vi "SubVI_Overlay Spot #.vi"(7 "Setup":T4={"Show Search Area"=FALSE, "Show Center"=FALSE, "Show Bounding Box"=TRUE}, 8 "Error in":errorcluster, 9 "Objects":T1(array[cluster]) {"Area" format="%.2f"; "Object Center"."Y" format="%.2f"; "Object Center"."X" format="%.2f"}, 10 "ROI":T3 {"Contours"."Type" items=["No Selection", "Point", "Line", "Rectangle", "Oval", "Polygon", "Free", "Annulus", "Unused2", "Unused3", "Broken Line", "Free Hand Line", "Rotated Rectangle"]}, 11 "Image In":T2) -> (0 "Error out":errorcluster, 3 "Image Out":T2)   [LabVIEW 2013]
uses:
  <vilib>/vision/Image Controls.llb/IMAQ Image.ctl
panel:
  in  "Center Color":u32(colorbox)=16711680
  in  "Search Area Color":u32(colorbox)=65280
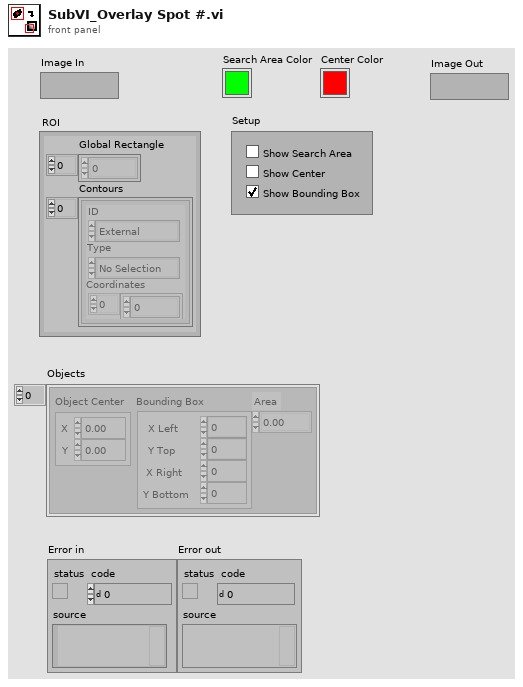
[diagram p1: front panel]
types:
  T1 = cluster{"Object Center":cluster{"X":dbl, "Y":dbl}, "Bounding Box":cluster{"X Left":dbl, "Y Top":dbl, "X Right":dbl, "Y Bottom":dbl}, "Area":dbl}[]
  T2 = typedef "IMAQ Image.ctl" = refnum<image>
  T3 = cluster{"Global Rectangle":i32[], "Contours":cluster{"ID":enum32{"External", "Internal"}, "Type":u32, "Coordinates":i32[]}[]}
  T4 = cluster{"Show Search Area":bool, "Show Center":bool, "Show Bounding Box":bool}
  T5 = cluster{"[0]":sgl, "[1]":sgl, "[2]":sgl, "[3]":sgl}
  T6 = cluster{"[0]":i32, "[1]":i32, "[2]":i32, "[3]":i32}
  T7 = cluster{"X Left":dbl, "Y Top":dbl, "X Right":dbl, "Y Bottom":dbl}
  T8 = cluster{"X Left":i32, "Y Top":i32, "X Right":i32, "Y Bottom":i32}
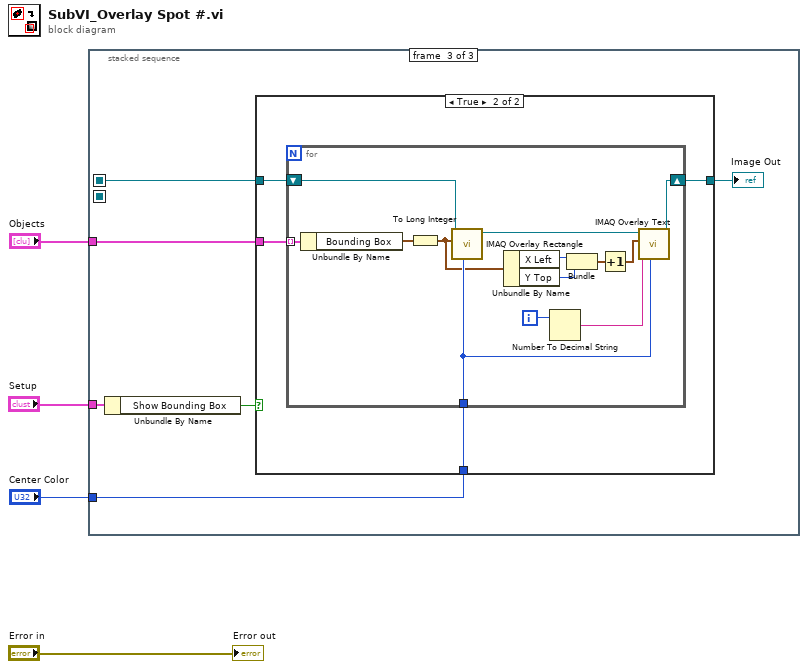
[diagram p0: block diagram]
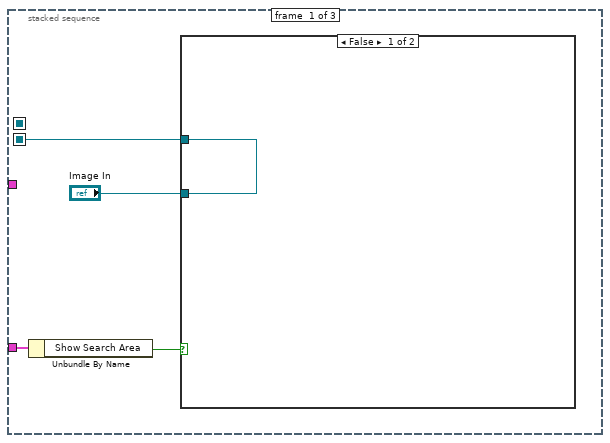
[diagram p2: hidden frame]
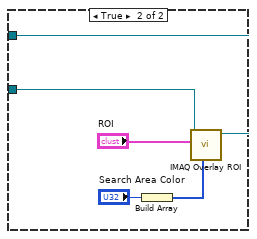
[diagram p3: hidden frame]
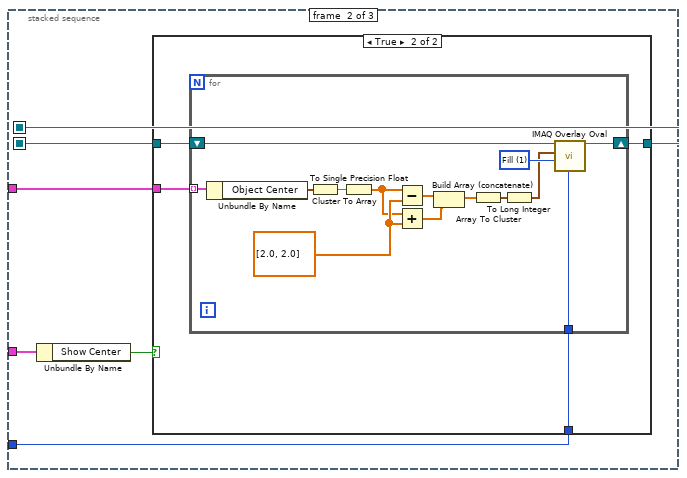
[diagram p4: hidden frame]
diagram:
  n1 = stacked-sequence {
    seq-local: [w5 _ _] -> [_ w20 _]
    seq-local: [_ w17 _] -> [_ _ w43]
    tunnel: "Setup" -> [w8 w16 w41]
    tunnel: "Objects" -> [_ w19 w45]
    tunnel: "Center Color" -> [_ w18 w42]
    frame #0 {
      n2 = Unbundle By Name(w8) -> ("Show Search Area"=w7:bool)
      n3 = case shown="False" w7 {
        tunnel: "Image In" -> [w9 w14]
        tunnel: [w9 w12] -> w5
        frame False {
        }
        frame True {
          n4 = Build Array("Search Area Color") -> (w10:u32[])
          n5 = call "IMAQ Overlay ROI"("Colors (Green)"=w10, "ROI Descriptor"="ROI", "Image"=w14) -> ("Image Out"=w12:T2)  [unwired: 3 in, 5 out]
        }
      }
    }
    frame #1 {
      n6 = Unbundle By Name(w16) -> ("Show Center"=w15:bool)
      n7 = case shown="True" w15 {
        tunnel: w20 -> [w21 w25]
        tunnel: w19 -> [_ w24]
        tunnel: w18 -> [_ w23]
        tunnel: [w21 w22] -> w17
        frame False {
        }
        frame True {
          n8 = for {
            shift-right: [w31] -> w22
            shift-left: w25 -> [w39]
            tunnel: w23 -> [w38]
            tunnel: w24 -> [w37] mode=indexing
            w30 = u32 1 items=["Frame", "Fill"] ("Drawing Mode (Frame)")
            w33 = sgl[] [2.0, 2.0] ("y")
            n9 = Unbundle By Name(w37) -> ("Object Center"=w32:cluster{"X":dbl, "Y":dbl})
            n10 = Cluster To Array(cluster=w32) -> (array=w29:dbl[])
            n11 = To Single Precision Float(number=w29) -> (single precision float=w28:sgl[])
            n12 = Subtract(x=w28, y=w33) -> (x-y=w36:sgl[])
            n13 = Add(x=w28, y=w33) -> (x+y=w35:sgl[])
            n14 = Build Array (concatenate)(w36, w35) -> (w34:sgl[])
            n15 = Array To Cluster(array=w34) -> (cluster=w27:T5)
            n16 = To Long Integer(number=w27) -> (32bit integer=w26:T6)
            n17 = call "IMAQ Overlay Oval"("Color"=w38, "Drawing Mode (Frame)"=w30, "Bounding Rectangle"=w26, "Image"=w39) -> ("Image Out"=w31:T2)  [unwired: 2 in, 5 out]
          }
        }
      }
    }
    frame #2 {
      n18 = Unbundle By Name(w41) -> ("Show Bounding Box"=w40:bool)
      n19 = case shown="True" w40 {
        tunnel: w45 -> [_ w50]
        tunnel: [w46 w49] -> w44
        tunnel: w43 -> [w46 w48]
        tunnel: w42 -> [_ w47]
        frame False {
        }
        frame True {
          n20 = for {
            shift-right: [w60] -> w49
            shift-left: w48 -> [w54]
            tunnel: w47 -> [w63]
            tunnel: w50 -> [w62] mode=indexing
            i -> [w61]
            n21 = Unbundle By Name(w62) -> ("Bounding Box"=w53:T7)
            n22 = To Long Integer(number=w53) -> (32bit integer=w51:T8)
            n23 = call "IMAQ Overlay Rectangle"("Color"=w63, "Rectangle"=w51, "Image"=w54) -> ("Image Out"=w58:T2)  [unwired: 3 in, 5 out]
            n24 = Unbundle By Name(w51) -> ("X Left"=w57:i32, "Y Top"=w56:i32)
            n25 = Number To Decimal String(number=w61) -> (decimal integer string=w59:string)  [unwired: 1 out]
            n26 = Bundle("X Left"=w57, "Y Top"=w56) -> (w55:cluster{"X Left":i32, "Y Top":i32})  [unwired: 1 out]
            n27 = Increment(x=w55) -> (x+1=w52:cluster{"X Left":i32, "Y Top":i32})
            n28 = call "IMAQ Overlay Text"("Text Color (black)"=w63, "String"=w59, "Origin"=w52, "Image"=w58) -> ("Image Out"=w60:T2)  [unwired: 4 in, 3 out]
          }
        }
      }
      "Image Out" <- w44
    }
  }
  "Error out" <- "Error in"
